vi "compare_frequency.vi"() -> ()   [LabVIEW 2020]
uses:
  common/record_file_handler/VFH-VNA_File_Handler.lvlib
panel:
  out "Waveform Graph 3":dbl[][](graph)
  out "Waveform Graph 2":dbl[][](graph)
  out "Waveform Graph":dbl[][](graph)
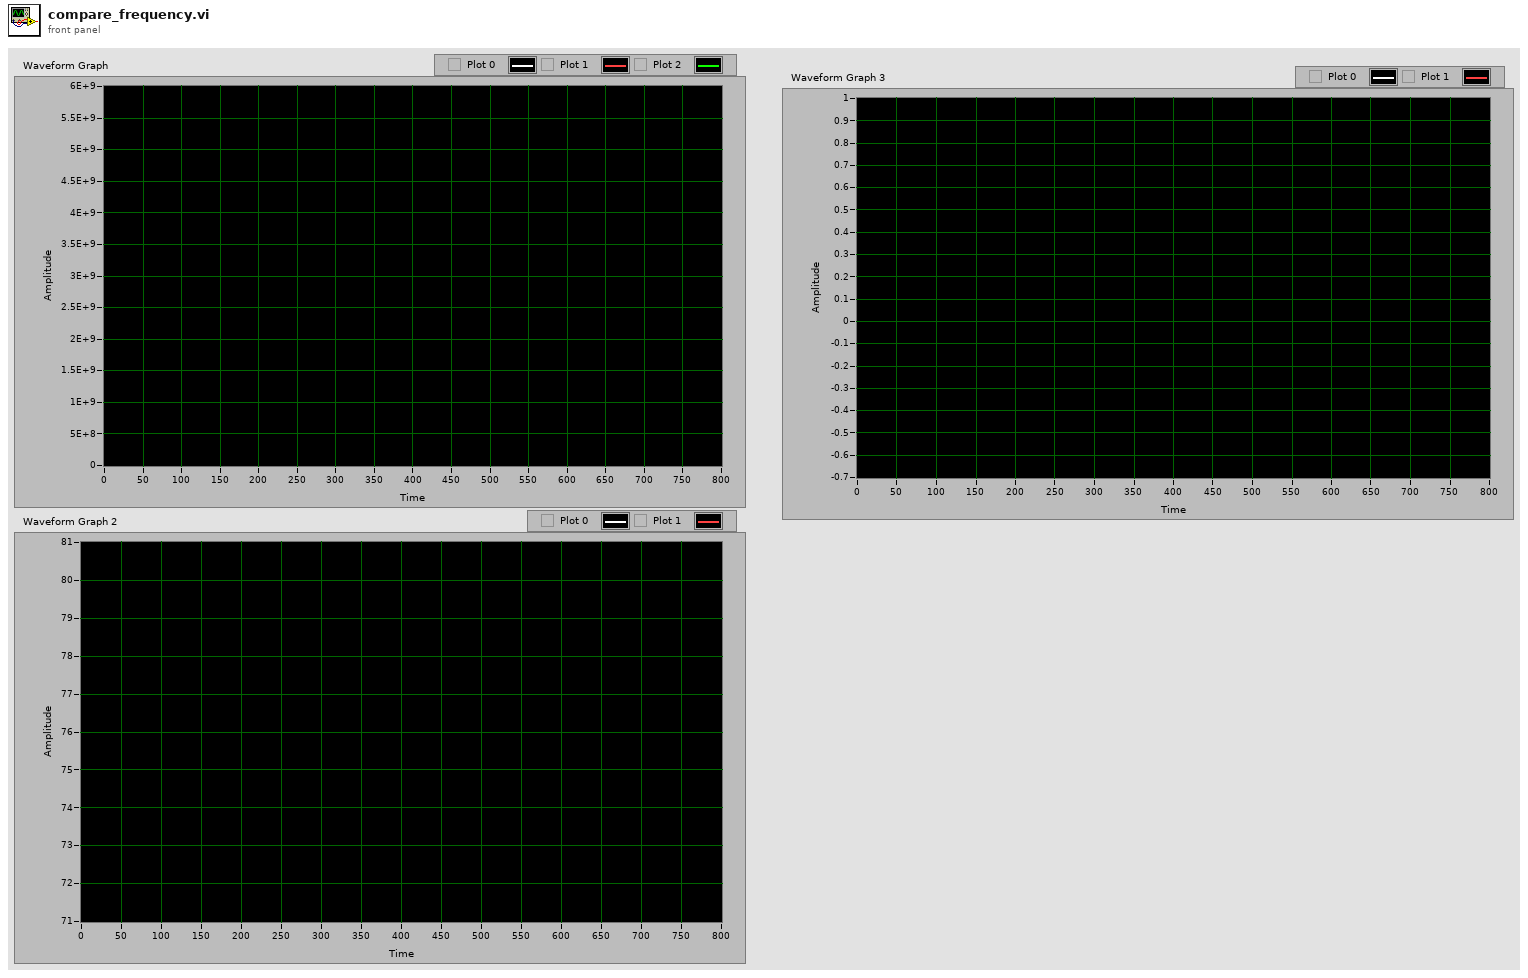
[diagram p1: front panel]
types:
  T1 = typedef "VFH-VNA_File_Handler.lvlib/VFH-file_cluster-NanoVNA.ctl" = cluster{"Frequency":dbl[], "S11_Real":dbl[], "S11_Imag":dbl[], "S21_Real":dbl[], "S21_Imag":dbl[], "S12_Real":dbl[], "S12_Imag":dbl[], "S22_Real":dbl[], "S22_Imag":dbl[]}
  T2 = typedef "VFH-VNA_File_Handler.lvlib/VFH-file_cluster-r140.ctl" = cluster{"Frequency":dbl[], "Permativity'":dbl[], "Permativity''":dbl[], "Q [S/m]":dbl[], "Tan":dbl[], "Reflection R":dbl[], "Reflection I":dbl[]}
  T3 = typedef "VFH-VNA_File_Handler.lvlib/VFH-file_cluster-r140_water.ctl" = cluster{"Frequency":dbl[], "Permativity'":dbl[], "Q [S/m]":dbl[]}
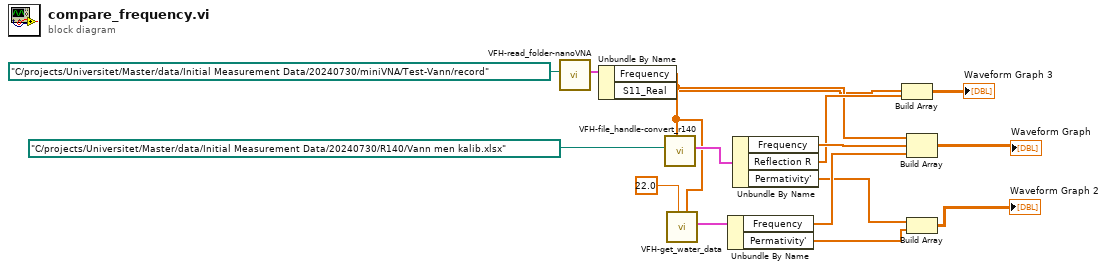
[diagram p0: block diagram]
diagram:
  n1 = call "VFH-read_folder-nanoVNA.vi"("Folder Path"=path "C:/projects/Universitet/Master/data/Initial Measurement Data/20240730/miniVNA/Test-Vann/record") -> ("avg output"=w13:T1)  [unwired: 8 in, 2 out]
  n2 = Unbundle By Name(w13) -> ("Frequency"=w6:dbl[], "S11_Real"=w1:dbl[])
  n3 = call "VFH-file_handle-convert_r140.vi"("Xi"=w6, "file path (dialog if empty)"=path "C:/projects/Universitet/Master/data/Initial Measurement Data/20240730/R140/Vann men kalib.xlsx") -> ("Handled data"=w12:T2)  [unwired: 9 in]
  n4 = call "VFH-get_water_data.vi"("Xi"=w6, "Water Temp"=22.0) -> ("Water Cluster"=w11:T3)  [unwired: 9 in]
  n5 = Unbundle By Name(w11) -> ("Frequency"=w9:dbl[], "Permativity'"=w3:dbl[])
  n6 = Unbundle By Name(w12) -> ("Frequency"=w10:dbl[], "Reflection R"=w7:dbl[], "Permativity'"=w4:dbl[])
  n7 = Build Array(w1, w7) -> (→"Waveform Graph 3":dbl[][])
  n8 = Build Array(w6, w10, w9) -> (→"Waveform Graph":dbl[][])
  n9 = Build Array(w4, w3) -> (→"Waveform Graph 2":dbl[][])
